vi "xiC - IMAQ - InitEventReg.vi"() -> (3 "EventRegRef":refnum<event-registration>)   [LabVIEW 2013]
uses:
  xiCamLib/xiLIB/xiC - Manager/xiCMNG - States.ctl
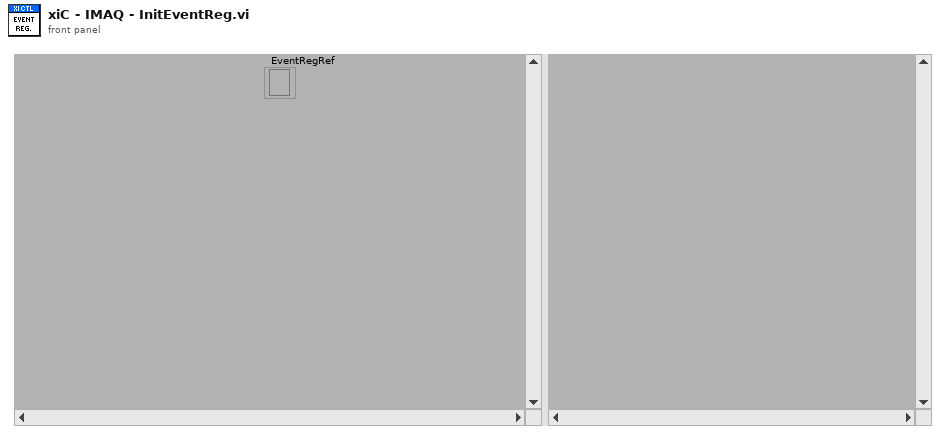
[diagram p1: front panel]
types:
  T1 = typedef "xiCMNG - States.ctl" = enum16{"Init", "Open", "Close", "Status"}
  T2 = typedef "xiCMNG - Attributes.ctl" = cluster{"VIPath":path, "VI Refnum":refnum<vi>, "SubPnl":refnum<vi>, "StopEvent":refnum<user-event>, "xiCam":refnum<k24>}
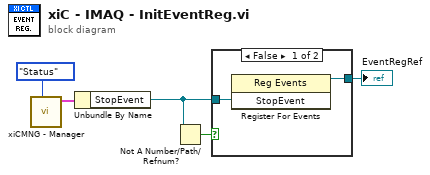
[diagram p0: block diagram]
diagram:
  n1 = call "xiCMNG - Manager.vi"("States"=xiCMNG_-_States."Status") -> ("StatusOut"=w4:T2)  [unwired: 9 in, 1 out]
  n2 = Unbundle By Name(w4) -> ("StopEvent"=w2:refnum<user-event>)
  n3 = Not A Number/Path/Refnum?(number/path/refnum=w2) -> (NaN/Path/Refnum?=w3:bool)
  n4 = case shown="False" w3 {
    tunnel: w2 -> [w7 _]
    tunnel: [w6 _] -> w1
    frame False {
      n5 = register-events(w7) -> (reference out=w6:refnum<event-registration>)  [unwired: 2 in, 1 out]
    }
    frame True {
    }
  }
  "EventRegRef" <- w1
